vi "Generic ROI Barycenter.vi"(8 "error in (no error)":errorcluster, 11 "ROI Descriptor":T1 {"Contours"."Type" items=["No Selection", "Point", "Line", "Rectangle", "Oval", "Polygon", "Freehand Region", "Annulus", "Unused2", "Unused3", "Broken Line", "Freehand Line", "Rotated Rectangle"]}) -> (0 "error out":errorcluster, 3 "ROI Center":cluster{"X":dbl, "Y":dbl})   [LabVIEW 2021, in "Image.lvlib"]
uses:
  Image.lvlib
  <vilib>/vision/NI_Vision_Development_Module.lvlib
  Error/Error.lvlib
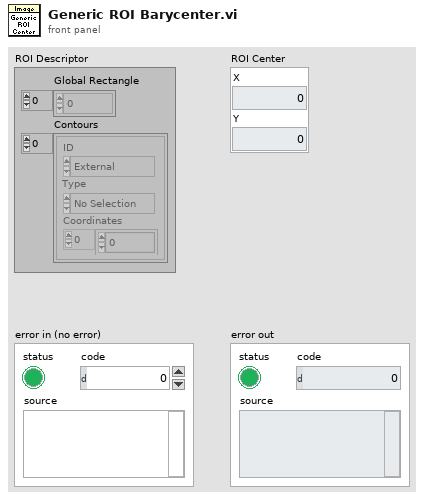
[diagram p1: front panel]
types:
  T1 = typedef "ROI Descriptor" = cluster{"Global Rectangle":i32[], "Contours":cluster{"ID":enum32{"External", "Internal"}, "Type":u32, "Coordinates":i32[]}[]}
  T2 = typedef "Image Type" = u32
  T3 = typedef "IMAQ Image.ctl" = refnum<image>
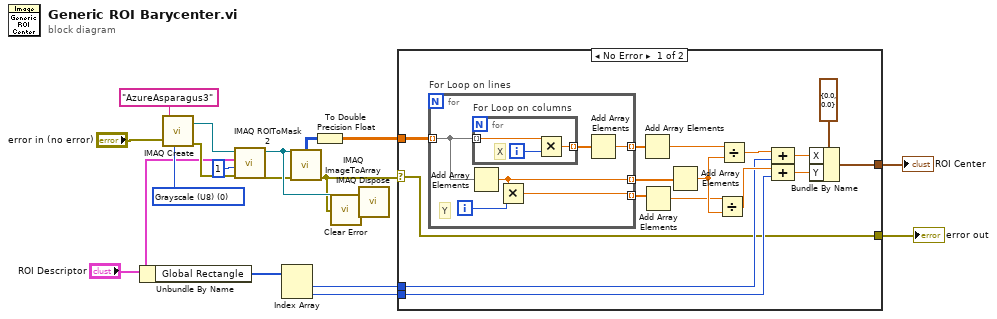
[diagram p0: block diagram]
diagram:
  w12 = T2 0 items=["Grayscale (U8)", "Grayscale (I16)", "Grayscale (SGL)", "Complex (CSG)", "RGB (U32)", "HSL (U32)", "RGB (U64)", "Grayscale (U16)"] ("Image Type")
  n1 = Unbundle By Name("ROI Descriptor") -> ("Global Rectangle"=w6:i32[])
  n2 = call "IMAQ Create"("Image Name"="AzureAsparagus3", "Image Type"=w12, "error in (no error)"="error in (no error)") -> ("New Image"=w9:T3, "error out"=w11:errorcluster)  [unwired: 2 in]
  n3 = call "IMAQ ROIToMask 2"("error in (no error)"=w11, "Filling Value (255)"=1, "ROI Descriptor"="ROI Descriptor", "Image"=w9) -> ("error out"=w14:errorcluster, "Image Out"=w15:T3)  [unwired: 5 in, 1 out]
  n4 = Index Array(array=w6) -> (element #1=w5:i32, element #2=w4:i32)  [unwired: 2 in]
  n5 = call "IMAQ ImageToArray"("error in (no error)"=w14, "Image"=w15) -> ("error out"=w3:errorcluster, "Image Pixels (U8)"=w16:u8[][])  [unwired: 2 in, 3 out]
  n6 = To Double Precision Float(number=w16) -> (double precision float=w17:dbl[][])
  n7 = call "Clear Error.vi"("Error In"=w3) -> ("no Error Out"=w1:errorcluster)  [unwired: 8 in]
  n8 = call "IMAQ Dispose"("Image"=w15, "error in (no error)"=w1) -> ()  [unwired: 4 in, 1 out]
  n9 = case shown="No Error" w3 {
    selector: w3 -> [w19 w44]
    tunnel: [w29 _] -> w18
    tunnel: w17 -> [w24 _]
    tunnel: w5 -> [w22 _]
    tunnel: w4 -> [w20 _]
    tunnel: [w19 w44] -> w2
    frame No Error {
      n10 = for "For Loop on lines" {
        tunnel: w24 -> [w37] mode=indexing
        tunnel: [w39] -> w26 mode=indexing
        tunnel: [w38] -> w25 mode=indexing
        tunnel: [w35] -> w31 mode=indexing
        i -> [w40]
        # "Y"
        n11 = Add Array Elements(numeric array=w37) -> (sum=w38:dbl)
        n12 = for "For Loop on columns" {
          tunnel: w37 -> [w43] mode=indexing
          tunnel: [w41] -> w36 mode=indexing
          i -> [w42]
          # "X"
          n13 = Multiply(x=w43, y=w42) -> (x*y=w41:dbl)
        }
        n14 = Multiply(x=w38, y=w40) -> (x*y=w39:dbl)
        n15 = Add Array Elements(numeric array=w36) -> (sum=w35:dbl)
      }
      n16 = Add Array Elements(numeric array=w31) -> (sum=w32:dbl)
      n17 = Add Array Elements(numeric array=w26) -> (sum=w27:dbl)
      n18 = Add Array Elements(numeric array=w25) -> (sum=w33:dbl)
      n19 = Divide(x=w27, y=w33) -> (x/y=w30:dbl)
      n20 = Divide(x=w32, y=w33) -> (x/y=w34:dbl)
      n21 = Compound Arithmetic op=ADD(w34, w22) -> (w23:dbl)
      n22 = Compound Arithmetic op=ADD(w30, w20) -> (w21:dbl)
      n23 = Bundle By Name(cluster=cluster{"X":dbl, "Y":dbl} {"X"=0.0, "Y"=0.0} ("ROI Center"), "X"=w23, "Y"=w21) -> (w29:cluster{"X":dbl, "Y":dbl})
    }
    frame Error {
    }
  }
  "ROI Center" <- w18
  "error out" <- w2
